vi "DAQ.vi"() -> ()   [LabVIEW 2015]
uses:
  globals.vi
  output_byte.vi
panel:
  out "In Drawing?":bool
  out "Shoulder":bool
  out "Elbow":bool
  out "Wrist":bool
  out "Motors Out":bool[](array[boolean])
  out "Switches In":bool[](array[boolean])
  out "shoulder angle":dbl
  out "Shoulder Angle":dbl(knob) scale=0.0..180.0
  out "Sh Max voltage":dbl
  out "Sh Min voltage":dbl
  out "Elbow Angle":dbl(knob) scale=0.0..180.0
  out "elbow angle":dbl
  out "El Max voltage":dbl
  out "El Min voltage":dbl
  in  "stop":bool
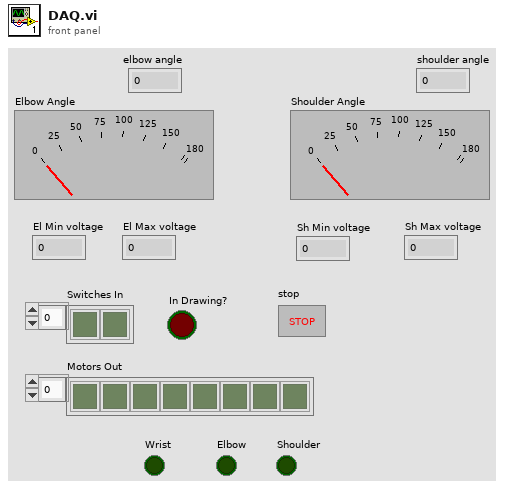
[diagram p1: front panel]
types:
  T1 = typedef "states.ctl" = enum16{"Idle", "Pause", "Next Contour", "Aligning", "Lowering Pen", "Drawing", "Next Point", "Lifting Pen", "Stop", "Put Away"}
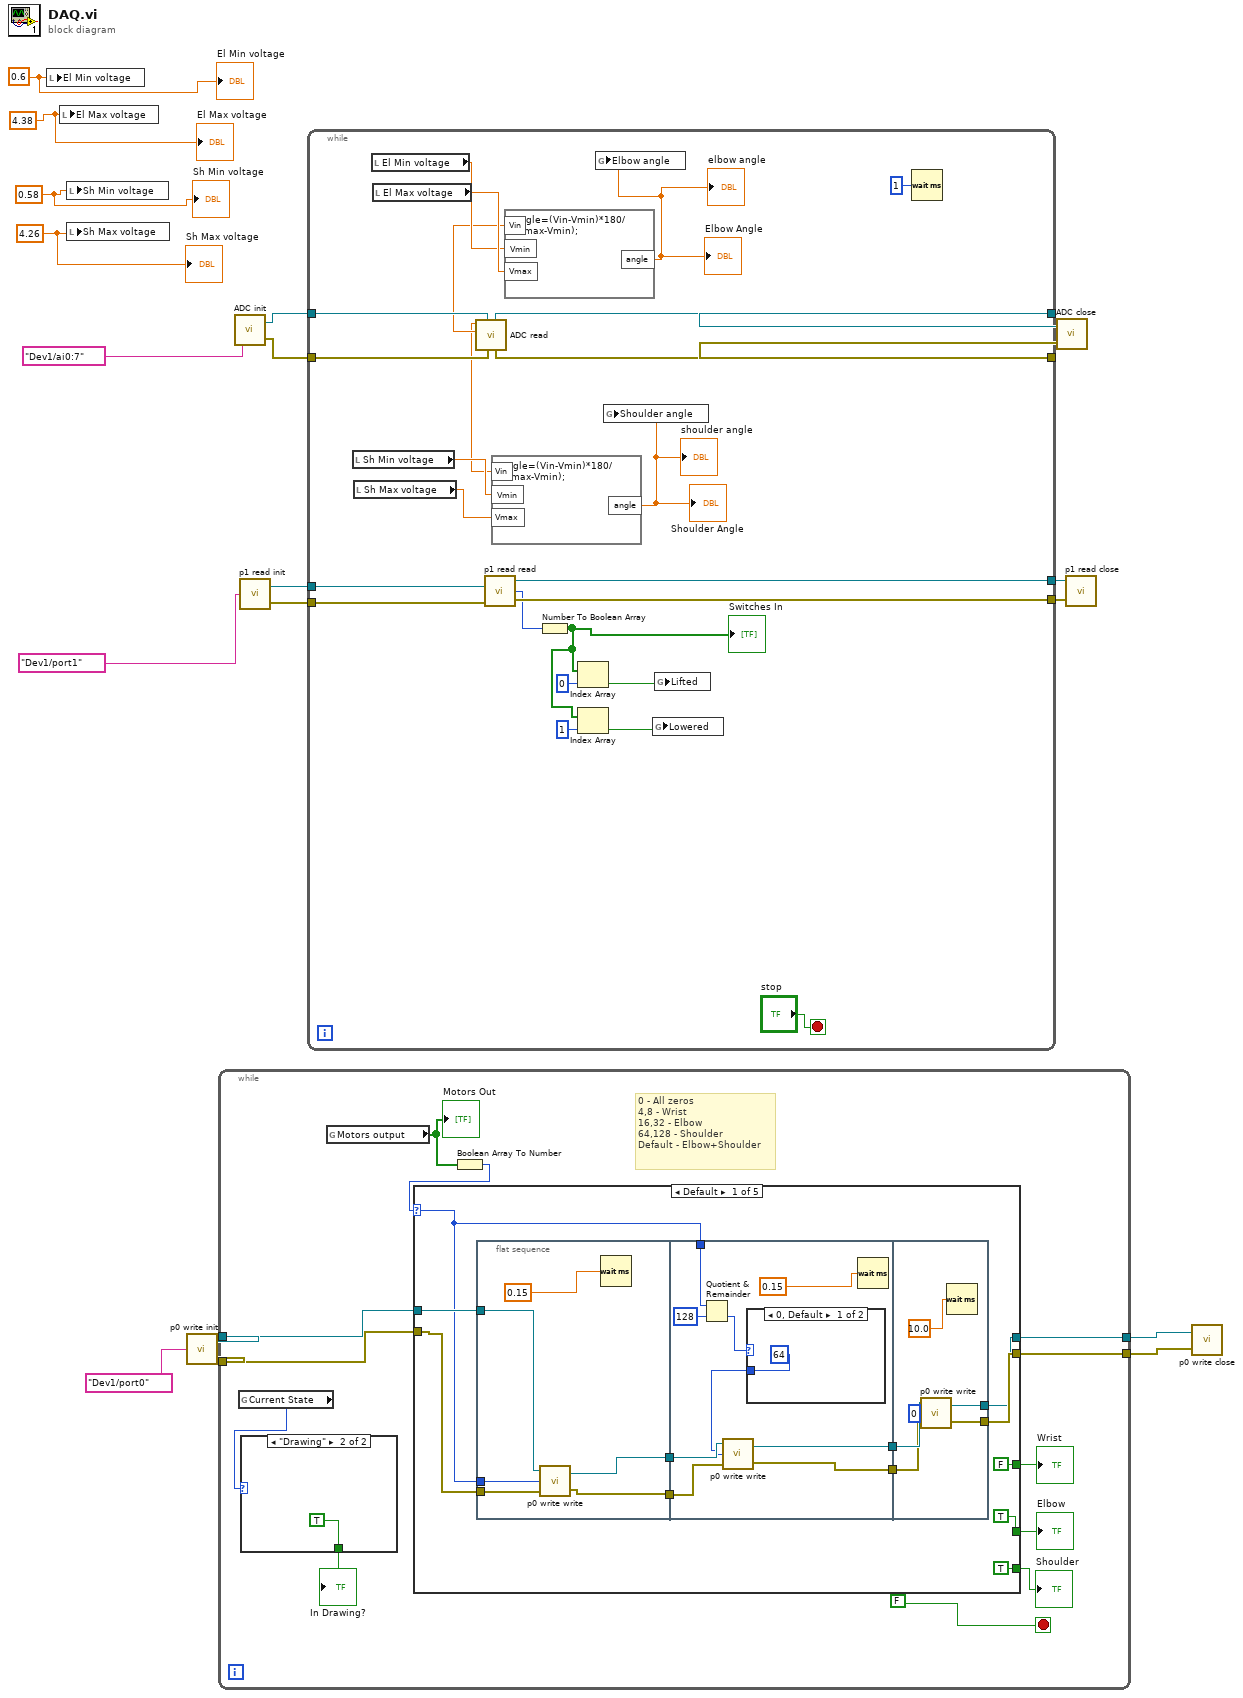
[diagram p0: block diagram]
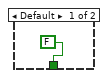
[diagram p2: hidden frame]
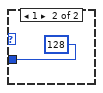
[diagram p3: hidden frame]
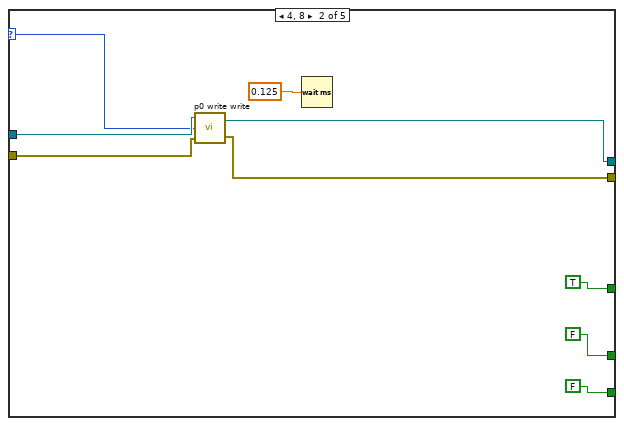
[diagram p4: hidden frame]
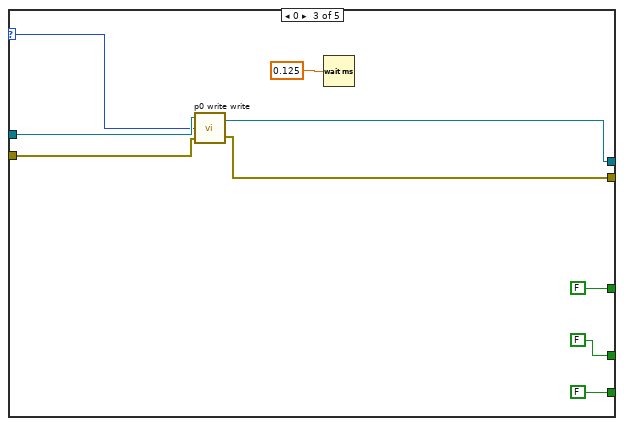
[diagram p5: hidden frame]
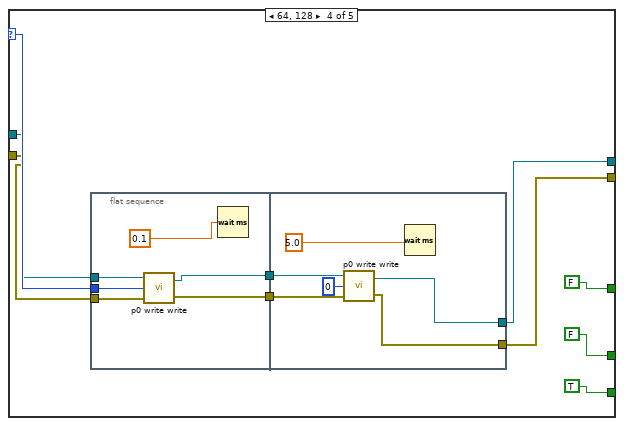
[diagram p6: hidden frame]
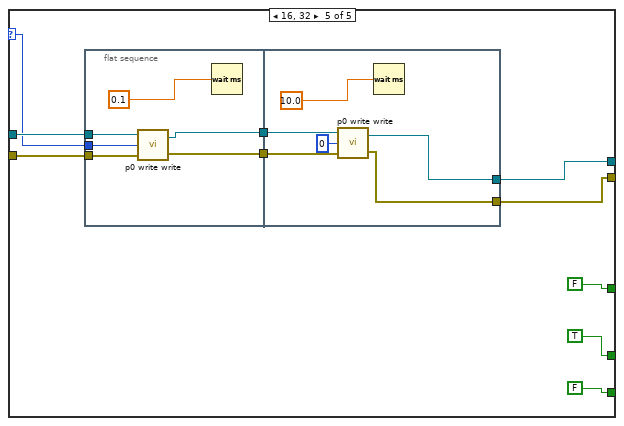
[diagram p7: hidden frame]
diagram:
  w11 = 4.26
  w12 = 0.58
  w14 = 4.38
  w13 = 0.6
  n1 = local write "El Min voltage"(w13) -> ()
  n2 = local write "El Max voltage"(w14) -> ()
  n3 = local write "Sh Min voltage"(w12) -> ()
  n4 = local write "Sh Max voltage"(w11) -> ()
  n5 = call "p0 write init.vi"("Port"=tag "Dev1/port0" ("Outputs (digital)")) -> ("task out"=w4:refnum<k21>, "error out"=w3:errorcluster)
  n6 = while {
    tunnel: w4 -> [w29]
    tunnel: w3 -> [w28]
    tunnel: [w26] -> w2
    tunnel: [w25] -> w1
    stop <- FALSE stop-if-true
    # "0 - All zeros\n4,8 - Wrist\n16,32 - Elbow\n64,128 - Shoulder\nDefault - Elbow+Shoulder"
    n7 = global read "output_byte.vi" "Current State"() -> (w21:T1)
    n8 = case shown="\"Drawing\"" w21 {
      tunnel: [FALSE TRUE] -> w20
      frame Default {
      }
      frame "Drawing" {
      }
    }
    "In Drawing?" <- w20
    n9 = global read "output_byte.vi" "Motors output"() -> (w31:bool[])
    "Motors Out" <- w31
    n10 = Boolean Array To Number(Boolean array=w31) -> (number=w27:u32)
    n11 = case shown="Default" w27 {
      selector: w27 -> [w41 w75 w84 w91 w114]
      tunnel: w29 -> [w43 w76 w85 w90 w116]
      tunnel: w28 -> [w42 w77 w86 w89 w115]
      tunnel: [w38 w73 w82 w87 w112] -> w26
      tunnel: [w37 w74 w83 w88 w113] -> w25
      tunnel: [FALSE TRUE FALSE FALSE FALSE] -> w24
      tunnel: [TRUE FALSE FALSE FALSE TRUE] -> w23
      tunnel: [TRUE FALSE FALSE TRUE FALSE] -> w22
      frame Default {
        n12 = flat-sequence {
          tunnel: [w51] -> w45
          tunnel: [w50] -> w44
          tunnel: w43 -> [w49]
          tunnel: w42 -> [w48]
          tunnel: w41 -> [w47]
          tunnel: w45 -> [w60]
          tunnel: w44 -> [w58]
          tunnel: w41 -> [w56]
          tunnel: [w59] -> w40
          tunnel: [w57] -> w39
          tunnel: w40 -> [w67]
          tunnel: w39 -> [w68]
          tunnel: [w66] -> w38
          tunnel: [w65] -> w37
          frame #0 {
            n13 = call "p0 write write.vi"("error in"=w48, "Data to Write"=w47, "task/channels in"=w49) -> ("error out"=w51:errorcluster, "task out"=w50:refnum<k21>)
            n14 = Wait (ms)(milliseconds to wait=0.15 ("Both")) -> ()  [unwired: 1 out]
          }
          frame #1 {
            n15 = Quotient & Remainder(x=w56, y=u32 128) -> (floor(x/y)=w54:u32)  [unwired: 1 out]
            n16 = case shown="0, Default" w54 {
              tunnel: [64 128] -> w53
              frame 0, Default {
              }
              frame 1 {
              }
            }
            n17 = call "p0 write write.vi"("error in"=w60, "Data to Write"=w53, "task/channels in"=w58) -> ("error out"=w59:errorcluster, "task out"=w57:refnum<k21>)
            n18 = Wait (ms)(milliseconds to wait=0.15 ("Only Shoulder")) -> ()  [unwired: 1 out]
          }
          frame #2 {
            n19 = call "p0 write write.vi"("error in"=w67, "Data to Write"=u32 0, "task/channels in"=w68) -> ("error out"=w66:errorcluster, "task out"=w65:refnum<k21>)
            n20 = Wait (ms)(milliseconds to wait=10.0 ("Wait3")) -> ()  [unwired: 1 out]
          }
        }
      }
      frame 4, 8 {
        n21 = call "p0 write write.vi"("error in"=w77, "Data to Write"=w75, "task/channels in"=w76) -> ("error out"=w73:errorcluster, "task out"=w74:refnum<k21>)
        n22 = Wait (ms)(milliseconds to wait=0.125 ("millisecond multiple")) -> ()  [unwired: 1 out]
      }
      frame 0 {
        n23 = call "p0 write write.vi"("error in"=w86, "Data to Write"=w84, "task/channels in"=w85) -> ("error out"=w82:errorcluster, "task out"=w83:refnum<k21>)
        n24 = Wait (ms)(milliseconds to wait=0.125 ("millisecond multiple")) -> ()  [unwired: 1 out]
      }
      frame 64, 128 {
        n25 = flat-sequence {
          tunnel: [w102] -> w93
          tunnel: [w101] -> w92
          tunnel: w91 -> [w100]
          tunnel: w90 -> [w99]
          tunnel: w89 -> [w98]
          tunnel: [w108] -> w88
          tunnel: w93 -> [w107]
          tunnel: w92 -> [w105]
          tunnel: [w104] -> w87
          frame #0 {
            n26 = call "p0 write write.vi"("error in"=w98, "Data to Write"=w100, "task/channels in"=w99) -> ("error out"=w101:errorcluster, "task out"=w102:refnum<k21>)
            n27 = Wait (ms)(milliseconds to wait=0.1 ("Shoulder")) -> ()  [unwired: 1 out]
          }
          frame #1 {
            n28 = call "p0 write write.vi"("error in"=w105, "Data to Write"=u32 0, "task/channels in"=w107) -> ("error out"=w104:errorcluster, "task out"=w108:refnum<k21>)
            n29 = Wait (ms)(milliseconds to wait=5.0 ("Wait2")) -> ()  [unwired: 1 out]
          }
        }
      }
      frame 16, 32 {
        n30 = flat-sequence {
          tunnel: w116 -> [w124]
          tunnel: w115 -> [w123]
          tunnel: [w122] -> w118
          tunnel: [w121] -> w117
          tunnel: w114 -> [w120]
          tunnel: [w130] -> w113
          tunnel: w118 -> [w129]
          tunnel: w117 -> [w127]
          tunnel: [w126] -> w112
          frame #0 {
            n31 = call "p0 write write.vi"("error in"=w123, "Data to Write"=w120, "task/channels in"=w124) -> ("error out"=w121:errorcluster, "task out"=w122:refnum<k21>)
            n32 = Wait (ms)(milliseconds to wait=0.1 ("Elbow")) -> ()  [unwired: 1 out]
          }
          frame #1 {
            n33 = call "p0 write write.vi"("error in"=w127, "Data to Write"=u32 0, "task/channels in"=w129) -> ("error out"=w126:errorcluster, "task out"=w130:refnum<k21>)
            n34 = Wait (ms)(milliseconds to wait=10.0 ("Wait1")) -> ()  [unwired: 1 out]
          }
        }
      }
    }
    "Wrist" <- w24
    "Elbow" <- w23
    "Shoulder" <- w22
  }
  n35 = call "ADC init.vi"("Physical Channel"=tag "Dev1/ai0:7" ("Potentiometers (ADC)")) -> ("task out"=w18:refnum<k21>, "error out"=w17:errorcluster)
  n36 = call "p1 read init.vi"("Port"=tag "Dev1/port1" ("Switches (digital)")) -> ("task out"=w7:refnum<k21>, "error out"=w9:errorcluster)
  n37 = while {
    tunnel: w18 -> [w154]
    tunnel: w17 -> [w153]
    tunnel: [w152] -> w16
    tunnel: [w151] -> w15
    tunnel: [w141] -> w10
    tunnel: w9 -> [w140]
    tunnel: w7 -> [w139]
    tunnel: [w138] -> w6
    stop <- "stop" stop-if-true
    n38 = local read "Sh Min voltage"() -> (w145:dbl)
    n39 = local read "Sh Max voltage"() -> (w144:dbl)
    n40 = local read "El Min voltage"() -> (w149:dbl)
    n41 = local read "El Max voltage"() -> (w150:dbl)
    n42 = call "ADC read.vi"("error in"=w153, "task/channels in"=w154) -> ("error out"=w151:errorcluster, "task out"=w152:refnum<k21>, "adc1"=w146:dbl, "adc0"=w143:dbl)  [unwired: 6 out]
    n43 = call "p1 read read.vi"("task in"=w139, "error in"=w140) -> ("task out"=w138:refnum<k21>, "Data Read"=w137:u32, "error out"=w141:errorcluster)
    n44 = formula code="angle=(Vin-Vmin)*180/(Vmax-Vmin);"("Vin"=w143, "Vmin"=w145, "Vmax"=w144) -> ("angle"=w142:dbl)
    "Shoulder Angle" <- w142
    "shoulder angle" <- w142
    n45 = formula code="angle=(Vin-Vmin)*180/(Vmax-Vmin);"("Vin"=w146, "Vmin"=w149, "Vmax"=w150) -> ("angle"=w148:dbl)
    "elbow angle" <- w148
    "Elbow Angle" <- w148
    n46 = Number To Boolean Array(number=w137) -> (Boolean array=w134:bool[])
    "Switches In" <- w134
    n47 = Index Array(array=w134, index=0) -> (element=w133:bool)
    n48 = Index Array(array=w134, index=1) -> (element=w132:bool)
    n49 = global write "globals.vi" "Elbow angle"(w148) -> ()
    n50 = global write "globals.vi" "Shoulder angle"(w142) -> ()
    n51 = global write "globals.vi" "Lowered"(w132) -> ()
    n52 = global write "globals.vi" "Lifted"(w133) -> ()
    n53 = Wait (ms)(milliseconds to wait=u32 1) -> ()  [unwired: 1 out]
  }
  n54 = call "ADC close.vi"("error in"=w15, "task/channels in"=w16) -> ()
  n55 = call "p1 read close.vi"("error in"=w10, "task in"=w6) -> ()
  n56 = call "p0 write close.vi"("error in"=w2, "task/channels in"=w1) -> ()
  "El Min voltage" <- w13
  "El Max voltage" <- w14
  "Sh Min voltage" <- w12
  "Sh Max voltage" <- w11
